vi "未命名 4 (子VI).vi"(10 "B":dbl, 11 "A":dbl) -> (1 "A*B":dbl, 2 "布尔":bool, 3 "A+B":dbl)   [LabVIEW 2012]
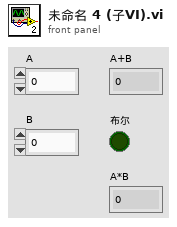
[diagram p1: front panel]
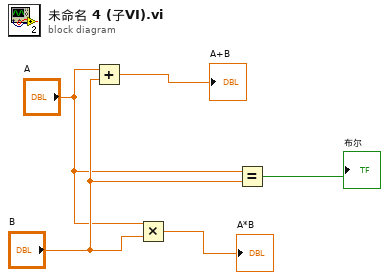
[diagram p0: block diagram]
diagram:
  n1 = Add(x="A", y="B") -> (x+y=→"A+B":dbl)
  n2 = Multiply(x="A", y="B") -> (x*y=→"A*B":dbl)
  n3 = Equal?(x="A", y="B") -> (x = y?=→"布尔":bool)
